vi "Read Test Case path.vi"(8 "error in (no error)":errorcluster, 10 "Test Case Name":string, 11 "Test Case Finder In":refnum<class "Test Finder.lvclass">) -> (0 "error out":errorcluster, 1 "found?":bool, 2 "Class path":path, 3 "Test Case Finder Out":refnum<class "Test Finder.lvclass">)   [LabVIEW 2020, in "Test Finder.lvclass"]
uses:
  Test Finder.lvclass
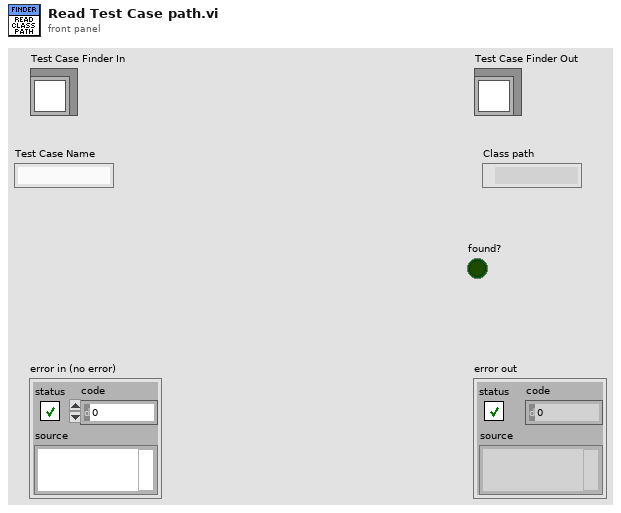
[diagram p1: front panel]
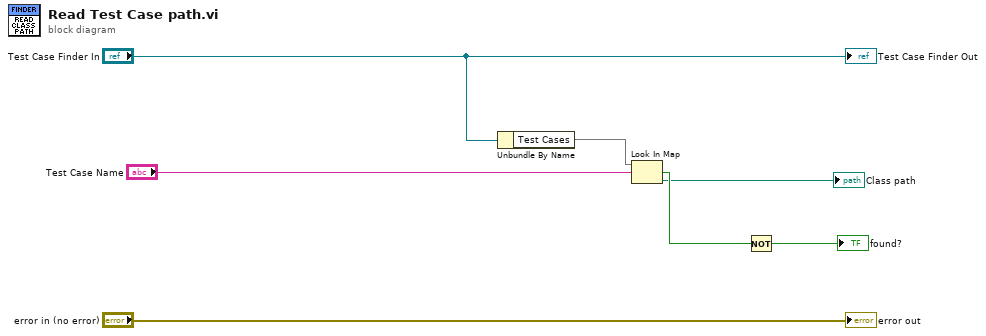
[diagram p0: block diagram]
diagram:
  n1 = Unbundle By Name("Test Case Finder In") -> ("Test Cases"=w5:map{string, path})
  n2 = Look In Map(map=w5, key="Test Case Name") -> (key not found?=w3:bool, value=→"Class path":path)  [unwired: 1 in]
  n3 = Not(x=w3) -> (.not. x?=→"found?":bool)
  "error out" <- "error in (no error)"
  "Test Case Finder Out" <- "Test Case Finder In"
